vi "slopes_processors_list_starter.vi"() -> ()   [LabVIEW 2018]
uses:
  Classes/HasoSlopes/HasoSlopes.lvclass
panel:
  in  "Output Haso slopes files base name":string="Data\\data_phase_computation_processed_"
  in  "Input Reference slopes file name":string="Data\\data_phase_computation.has"
  in  "Input Haso slopes files base name":string="Data\\data_phase_computation_"
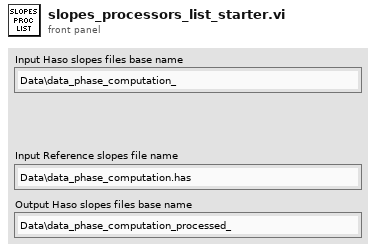
[diagram p1: front panel]
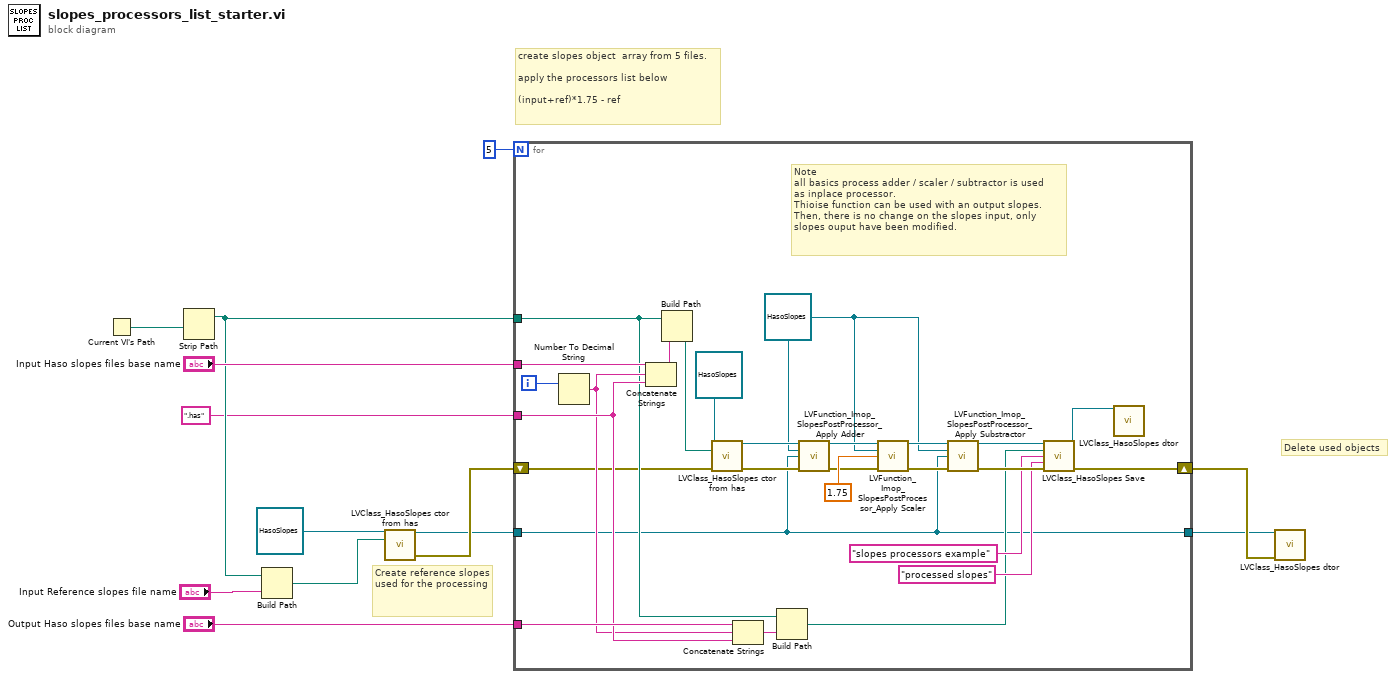
[diagram p0: block diagram]
diagram:
  # "Delete used objects"
  # "Create reference slopes used for the processing"
  # "create slopes object  array from 5 files.\n\napply the processors list below\n\n(input+ref)*1.75 - ref"
  n1 = Current VI's Path() -> (path=w12:path)
  n2 = Strip Path(path=w12) -> (stripped path=w8:path)  [unwired: 1 out]
  n3 = Build Path(base path=w8, name or relative path="Input Reference slopes file name") -> (appended path=w10:path)
  n4 = call "LVClass_HasoSlopes ctor from has.vi"("HasoSlopes (const)"=refnum<class "HasoSlopes.lvclass"> refnum ("HasoSlopes in"), ".has path"=w10) -> ("HasoSlopes (new)"=w3:refnum<class "HasoSlopes.lvclass">, "error out"=w4:errorcluster)  [unwired: 12 in]
  n5 = for {
    N: 5 -> [_]
    tunnel: w8 -> [w34]
    shift-right: [w19] -> w2
    shift-left: w4 -> [w31]
    tunnel: ".has" ("Haso slopes files extension") -> [w36]
    tunnel: "Input Haso slopes files base name" -> [w38]
    tunnel: "Output Haso slopes files base name" -> [w37]
    tunnel: w3 -> [w15]
    tunnel: [w15] -> w1
    i -> [w40]
    w14 = refnum<class "HasoSlopes.lvclass"> refnum ("HasoSlopes in")
    # "Note\nall basics process adder / scaler / subtractor is used\nas inplace processor. \nThioise function can be used with an output slopes.\nThen, there is no change on the slopes input, only\nslopes ouput have been modified."
    n6 = Number To Decimal String(number=w40) -> (decimal integer string=w35:string)  [unwired: 1 in]
    n7 = Concatenate Strings(w38, w35, w36) -> (w39:string)
    n8 = Build Path(base path=w34, name or relative path=w39) -> (appended path=w32:path)
    n9 = call "LVClass_HasoSlopes ctor from has.vi"("HasoSlopes (const)"=refnum<class "HasoSlopes.lvclass"> refnum ("HasoSlopes in"), ".has path"=w32, "error in (no error)"=w31) -> ("HasoSlopes (new)"=w29:refnum<class "HasoSlopes.lvclass">, "error out"=w20:errorcluster)  [unwired: 11 in]
    n10 = Concatenate Strings(w37, w35, w36) -> (w33:string)
    n11 = Build Path(base path=w34, name or relative path=w33) -> (appended path=w16:path)
    n12 = call "LVFunction_Imop_SlopesPostProcessor_Apply Adder.vi"("HasoSlopes in"=w29, "HasoSlopes OUT"=w14, "HasoSlopes to add"=w15, "error in (no error)"=w20) -> ("HasoSlopes out"=w27:refnum<class "HasoSlopes.lvclass">, "error out"=w25:errorcluster)  [unwired: 9 in, 1 out]
    n13 = call "LVFunction_Imop_SlopesPostProcessor_Apply Scaler.vi"("HasoSlopes in"=w27, "HasoSlopes OUT"=w14, "Scaler"=sgl 1.75 ("scaler"), "error in (no error)"=w25) -> ("HasoSlopes out"=w26:refnum<class "HasoSlopes.lvclass">, "error out"=w24:errorcluster)  [unwired: 9 in, 1 out]
    n14 = call "LVFunction_Imop_SlopesPostProcessor_Apply Substractor.vi"("HasoSlopes in"=w26, "HasoSlopes OUT"=w14, "HasoSlopes to substract"=w15, "error in (no error)"=w24) -> ("HasoSlopes out"=w21:refnum<class "HasoSlopes.lvclass">, "error out"=w23:errorcluster)  [unwired: 9 in, 1 out]
    n15 = call "LVClass_HasoSlopes Save.vi"("HasoSlopes in"=w21, "path"=w16, "comments"="slopes processors example", "session"="processed slopes", "error in (no error)"=w23) -> ("HasoSlopes out"=w22:refnum<class "HasoSlopes.lvclass">, "error out"=w19:errorcluster)  [unwired: 9 in]
    n16 = call "LVClass_HasoSlopes dtor.vi"("HasoSlopes in"=w22) -> ()  [unwired: 13 in, 2 out]
  }
  n17 = call "LVClass_HasoSlopes dtor.vi"("HasoSlopes in"=w1, "error in (no error)"=w2) -> ()  [unwired: 12 in, 2 out]
